vi "receive.vi"(8 "error in (no error)":errorcluster, 10 "Data":u16[](array[numeric]), 11 "Modbus in":refnum<class "Modbus.lvclass">) -> (0 "error out":errorcluster, 2 "RxFrame":T1 {"Data" format="%02x"}, 3 "Modbus out":refnum<class "Modbus.lvclass">)   [LabVIEW 2016, in "RTModbusFPGA.lvlib" / "Modbus.lvclass"]
uses:
  Modbus.lvclass
  DataTypes/RxFrame.ctl
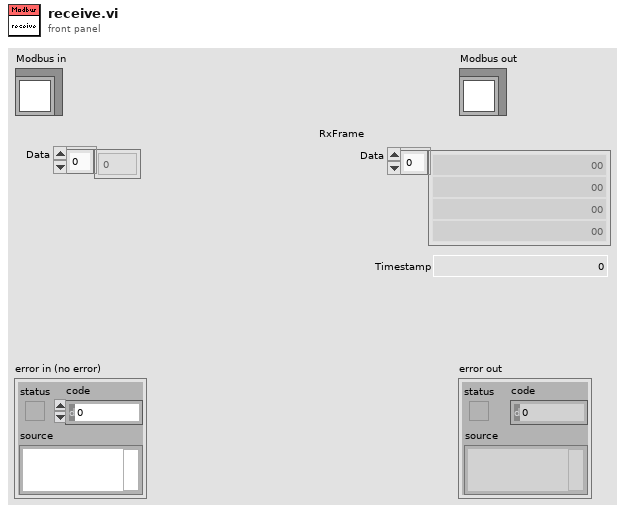
[diagram p1: front panel]
types:
  T1 = typedef "RxFrame.ctl" = cluster{"Data":u8[], "Timestamp":u64}
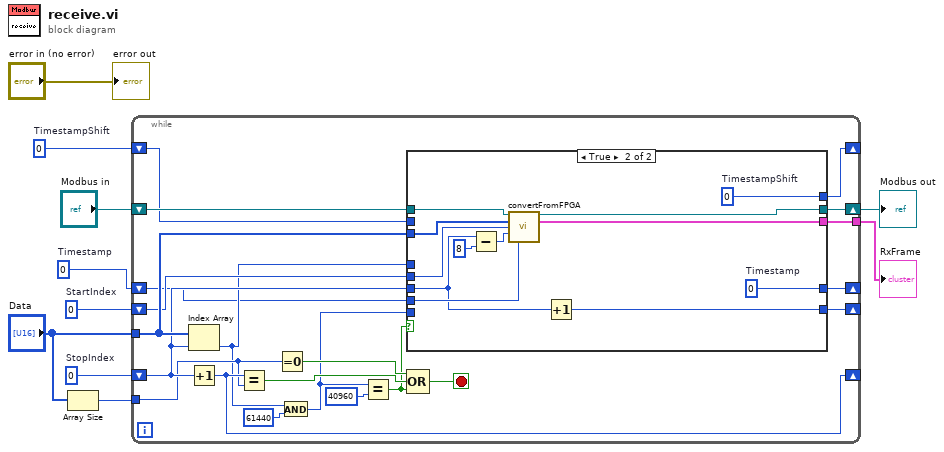
[diagram p0: block diagram]
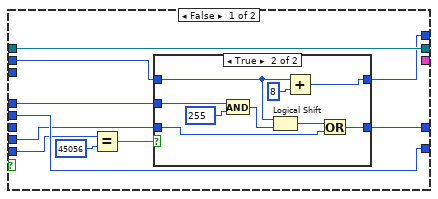
[diagram p2: hidden frame]
diagram:
  w4 = 0  # TimestampShift
  w5 = u64 0  # Timestamp
  w7 = 0  # StartIndex
  w8 = 0  # StopIndex
  n1 = Array Size(array="Data") -> (size(s)=w6:i32)
  n2 = while {
    shift-right: [w29] -> _
    shift-left: w8 -> [w25]
    shift-right: [w24] -> _
    shift-left: w7 -> [w26]
    tunnel: "Data" -> [w27]
    tunnel: w6 -> [w22]
    shift-right: [w23] -> w2
    shift-left: "Modbus in" -> [w28]
    shift-right: [w17] -> _
    shift-left: w5 -> [w16]
    shift-right: [w14] -> _
    shift-left: w4 -> [w15]
    tunnel: [w13] -> w1
    stop <- w11 stop-if-true
    n3 = Index Array(array=w27, index=w25) -> (element=w18:u16)
    n4 = Increment(x=w25) -> (x+1=w29:i32)
    n5 = Equal?(x=w29, y=w22) -> (x = y?=w20:bool)
    n6 = Equal To 0?(x=w22) -> (x = 0?=w21:bool)
    n7 = And(x=w18, y=u16 61440) -> (x .and. y?=w19:u16)
    n8 = Equal?(x=w19, y=u16 40960) -> (x = y?=w12:bool)
    n9 = case shown="True" w12 {
      tunnel: w28 -> [w40 w64]
      tunnel: w27 -> [_ w63]
      tunnel: w26 -> [w41 w62]
      tunnel: w25 -> [_ w57]
      tunnel: [w41 w60] -> w24
      tunnel: [w40 w61] -> w23
      tunnel: w19 -> [w39 _]
      tunnel: w18 -> [w36 _]
      tunnel: [w34 w59] -> w17
      tunnel: w16 -> [w35 w58]
      tunnel: w15 -> [w33 _]
      tunnel: [w32 w54] -> w14
      tunnel: [_ w53] -> w13
      frame False {
        n10 = Equal?(x=w39, y=u16 45056) -> (x = y?=w37:bool)
        n11 = case shown="True" w37 {
          tunnel: w36 -> [_ w52]
          tunnel: w35 -> [w43 w47]
          tunnel: [w43 w48] -> w34
          tunnel: w33 -> [w42 w46]
          tunnel: [w42 w44] -> w32
          frame False {
          }
          frame True {
            n12 = And(x=w52, y=u64 255) -> (x .and. y?=w49:u64)
            n13 = Logical Shift(y=w46, x=w49) -> (x << y=w50:u64)
            n14 = Add(x=w46, y=8) -> (x+y=w44:i32)
            n15 = Or(x=w50, y=w47) -> (x .or. y?=w48:u64)
          }
        }
      }
      frame True {
        w54 = 0  # TimestampShift
        w59 = u64 0  # Timestamp
        n16 = Subtract(x=w57, y=8) -> (x-y=w55:i32)
        n17 = call "convertFromFPGA.vi"("Modbus in"=w64, "Data"=w63, "StartIndex"=w62, "StopIndex"=w55, "Timestamp"=w58) -> ("Modbus out"=w61:refnum<class "Modbus.lvclass">, "RxFrame"=w53:T1)  [unwired: 8 in, 1 out]
        n18 = Increment(x=w57) -> (x+1=w60:i32)
      }
    }
    n19 = Compound Arithmetic op=OR(w21, w20, w12) -> (w11:bool)
  }
  "Modbus out" <- w2
  "RxFrame" <- w1
  "error out" <- "error in (no error)"
